vi "Y[i]=Clip{X[i]} PtByPt.vi"(2 "lower limit":dbl format="%0.2f", 3 "upper limit":dbl=1.0 format="%0.2f", 4 "x":dbl format="%0.2f") -> (0 "error":i32, 1 "clipped x":dbl format="%0.2f")   [LabVIEW 2017, in "NI_PtbyPt.lvlib"]
doc: "Clips <B>x</B> to within the bounds specified by <B>upper limit</B> and <B>lower limit</B>."
uses:
  <vilib>/ptbypt/NI_PtbyPt.lvlib
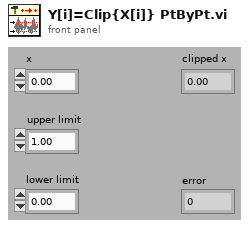
[diagram p1: front panel]
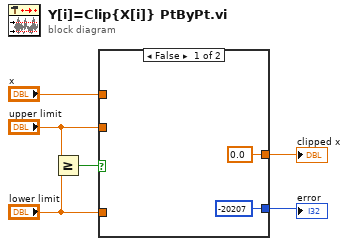
[diagram p0: block diagram]
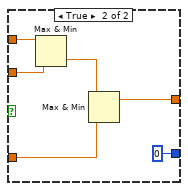
[diagram p2: hidden frame]
diagram:
  n1 = Greater Or Equal?(x="upper limit", y="lower limit") -> (x >= y?=w2:bool)
  n2 = case shown="False" w2 {
    tunnel: "x" -> [_ w14]
    tunnel: "upper limit" -> [_ w13]
    tunnel: "lower limit" -> [_ w12]
    tunnel: [0.0 ("lower limit") w10] -> w5
    tunnel: [-20207 ("error") 0 ("error")] -> w1
    frame False {
    }
    frame True {
      n3 = Max & Min(x=w14, y=w13) -> (min(x,y)=w11:dbl)  [unwired: 1 out]
      n4 = Max & Min(x=w11, y=w12) -> (max(x,y)=w10:dbl)  [unwired: 1 out]
    }
  }
  "clipped x" <- w5
  "error" <- w1
